vi "Test SenseHat Basic.vi"() -> ()   [LabVIEW 2020]
uses:
  src/RPI.SenseHat/SenseHat/SenseHat.lvclass/SenseHat.ctl
  src/RPI.SenseHat/SenseHat/Get RPI.SenseHat.Joystick.vi
  src/RPI.SenseHat/SenseHat/Get RPI.SenseHat.Display.vi
  tests/RPI.SenseHat_Tests/Arrows.vi
  src/RPI.SenseHat.Joystick/Classes/senseHatJoystick/RPI.SenseHat.Joystick.lvclass
  src/RPI.SenseHat.Display/Classes/SenseHat.Display/RPI.SenseHat.Display.lvclass
  <vilib>/MakerHub/LINX/Public/Utilities/Open Local.vi
  <vilib>/MakerHub/LINX/LMH-LINX.lvlib
  src/RPI.SenseHat/SenseHat/SenseHat.lvclass
  src/RPI.SenseHat.Display/RPI.SenseHat.Display.lvlib
panel:
  out "s? t:f":u32[][](array[colorbox])
  in  "Stop":bool
  out "Device Name":string
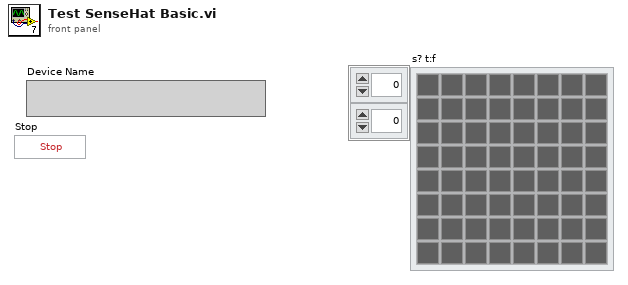
[diagram p1: front panel]
types:
  T1 = typedef "LMH-LINX.lvlib/LINX Ref.ctl" = cluster{"IO":T2, "Interface":T3, "LINX Device Config":T4}
  T2 = typedef "LMH-LINX.lvlib/Platform.ctl" = enum16{"Remote", "Local"}
  T3 = typedef "LMH-LINX.lvlib/Interface.ctl" = enum16{"Serial", "TCP"}
  T4 = typedef "LMH-LINX.lvlib/Device.lvlib/LINX Device Config.ctl" = cluster{"Interface":T3, "COM Port":refnum<visa-resource-name>, "TCP Configuration":T5, "Device Family":u8, "Device ID":u8, "Device Name":string, "TCP Ref":refnum<k5>, "Channels":T6}
  T5 = typedef "LMH-LINX.lvlib/Device.lvlib/TCP Config.ctl" = cluster{"IP Address":string, "Port":u16}
  T6 = typedef "LMH-LINX.lvlib/Channels.ctl" = cluster{"DI":u8[], "DO":u8[], "AI":u8[], "AO":u8[], "PWM":u8[], "QE":u8[], "UART":u8[], "I2C 2":u8[], "SPI":u8[], "CAN":u8[], "Servo":u8[], "AI Ref (V)":dbl, "AI Resolution (Bits)":u8, "AO Ref (V)":dbl, "AO Resolution (Bits)":u8}
  T7 = typedef "RPI.SenseHat.Joystick.lvlib/Joystick.ctl" = cluster{"Enter":bool, "Down":bool, "Up":bool, "Right":bool, "Left":bool}
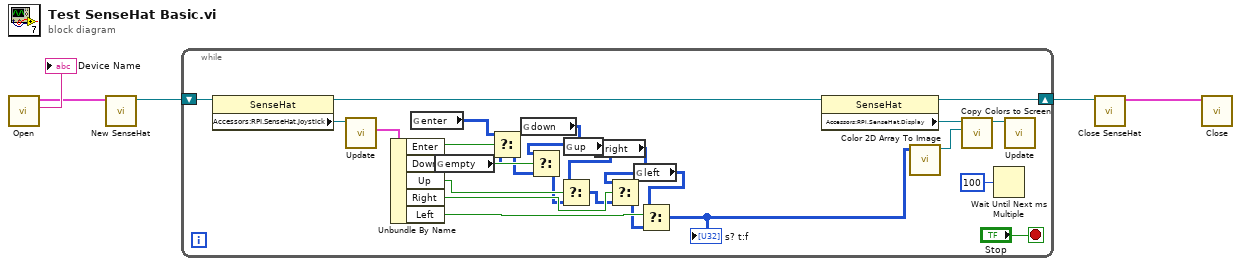
[diagram p0: block diagram]
diagram:
  n1 = call-poly <vilib>:"Open.vi"() -> ("Device Name"=→"Device Name":string, "LINX Resource"=w4:T1)  [unwired: 9 in, 1 out]
  n2 = call "New SenseHat.vi"("LINX Resource"=w4) -> ("SenseHat out"=w2:refnum<class "SenseHat.lvclass">)  [unwired: 9 in, 1 out]
  n3 = while {
    shift-right: [w27] -> w1
    shift-left: w2 -> [w30]
    stop <- "Stop" stop-if-true
    n4 = property class="SenseHat"(reference=w30) -> (reference out=w29:refnum<class "SenseHat.lvclass">, "Accessors:RPI.SenseHat.Joystick"=w31:refnum<class "RPI.SenseHat.Joystick.lvclass">)  [unwired: 1 in, 1 out]
    n5 = call "Update.vi"("senseHatJoystick in"=w31) -> ("Joystick"=w23:T7)  [unwired: 8 in, 2 out]
    n6 = Unbundle By Name(w23) -> ("Enter"=w22:bool, "Down"=w20:bool, "Up"=w18:bool, "Right"=w15:bool, "Left"=w14:bool)
    n7 = global read "Arrows.vi" "enter"() -> (w21:u32[][])
    n8 = global read "Arrows.vi" "empty"() -> (w8:u32[][])
    n9 = Select(t=w21, s=w22, f=w8) -> (s? t:f=w9:u32[][])
    n10 = global read "Arrows.vi" "down"() -> (w19:u32[][])
    n11 = Select(t=w19, s=w20, f=w9) -> (s? t:f=w10:u32[][])
    n12 = global read "Arrows.vi" "up"() -> (w17:u32[][])
    n13 = Select(t=w17, s=w18, f=w10) -> (s? t:f=w11:u32[][])
    n14 = global read "Arrows.vi" "right"() -> (w16:u32[][])
    n15 = Select(t=w16, s=w15, f=w11) -> (s? t:f=w12:u32[][])
    n16 = global read "Arrows.vi" "left"() -> (w13:u32[][])
    n17 = Select(t=w13, s=w14, f=w12) -> (s? t:f=w7:u32[][])
    "s? t:f" <- w7
    n18 = property class="SenseHat"(reference=w29) -> (reference out=w27:refnum<class "SenseHat.lvclass">, "Accessors:RPI.SenseHat.Display"=w28:refnum<class "RPI.SenseHat.Display.lvclass">)  [unwired: 1 in, 1 out]
    n19 = call "Color 2D Array To Image.vi"("Color[]"=w7) -> ("Image out"=w26:refnum<class "Image.lvclass">)  [unwired: 9 in, 1 out]
    n20 = call "Copy Colors to Screen.vi"("Image"=w26, "senseHatDisplay in"=w28) -> ("senseHatDisplay out"=w6:refnum<class "RPI.SenseHat.Display.lvclass">)  [unwired: 8 in, 1 out]
    n21 = Wait Until Next ms Multiple(millisecond multiple=u32 100) -> ()  [unwired: 1 out]
    n22 = call "Update.vi"("senseHatDisplay in"=w6) -> ()  [unwired: 9 in, 2 out]
  }
  n23 = call "Close SenseHat.vi"("SenseHat in"=w1) -> ("LINX Resource"=w3:T1)  [unwired: 9 in, 1 out]
  n24 = call <vilib>:"Close.vi"("LINX Resource"=w3) -> ()  [unwired: 10 in, 1 out]
